vi "user32_ReleaseCapture.vi"(8 "错误输入（无错误）":errorcluster, 11 "路径输入":path) -> (0 "错误输出":errorcluster, 2 "返回值":i32, 3 "路径输出":path)   [LabVIEW 2017]
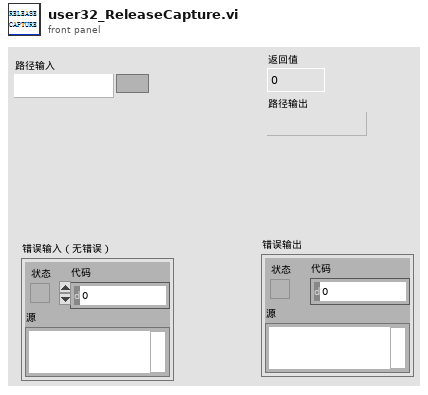
[diagram p1: front panel]
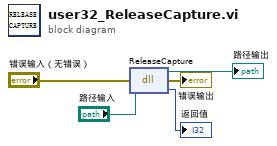
[diagram p0: block diagram]
diagram:
  n1 = dll-call lib="C:/Windows/System32/user32.dll" fn="ReleaseCapture"(path in="路径输入", error in="错误输入（无错误）") -> (path out=→"路径输出":path, error out=→"错误输出":errorcluster, "返回值"=→"返回值":i32)  [unwired: 1 in]
